vi "Analog Replay 1.0 In Place Input Write Structure.vi"(5 "Device Inputs":dbl[](array[numeric]), 7 "Last Device Inputs":dbl[](array[numeric]), 8 "error in (no error)":errorcluster, 10 "Refnum in":T3, 11 "1.0.0 Analog Replay in":T1) -> (0 "error out":errorcluster, 2 "Refnum out":T3, 3 "1.0.0 Analog Replay out":T1)   [LabVIEW 2013, in "Engine Simulation Toolkit Engine.lvlib"]
uses:
  Engine Simulation Toolkit Engine.lvlib
  Analog Replay 1.0 Input Ref.ctl
  Shared/1.0 Analog Replay Engine Data.ctl
  Shared/1.0 Analog Replay FIFO Idxs.ctl
  Shared/Engine Simulation Toolkit Shared.lvlib
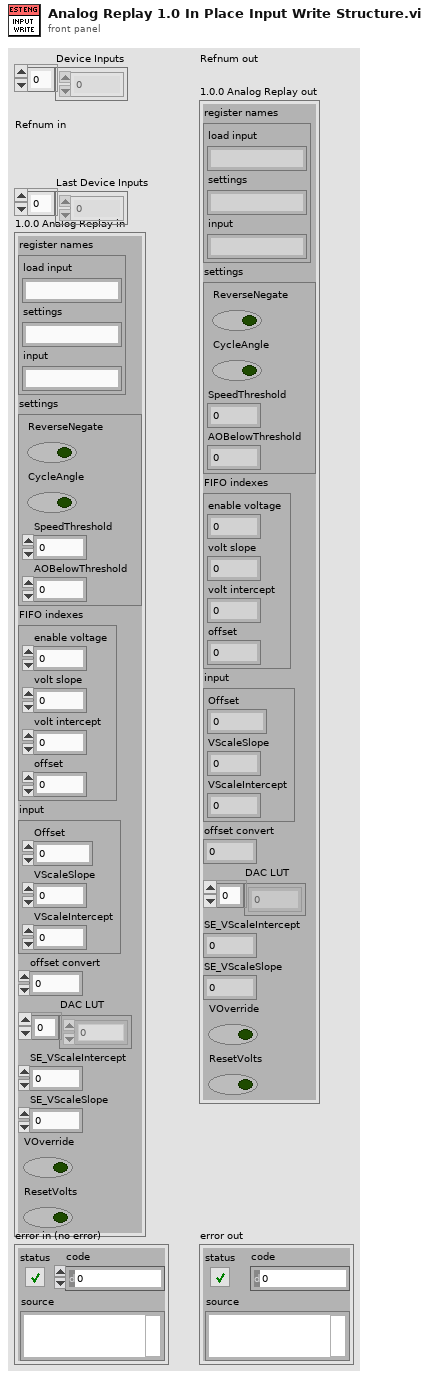
[diagram p1: front panel]
types:
  T1 = typedef "Engine Simulation Toolkit Shared.lvlib/1.0 Analog Replay Engine Data.ctl" = cluster{"register names":cluster{"load input":string, "settings":string, "input":string}, "settings":cluster{"ReverseNegate":bool, "CycleAngle":bool, "SpeedThreshold":fxp<+/-,23,2>, "AOBelowThreshold":i16}, "FIFO indexes":T2, "input":cluster{"Offset":i16, "VScaleSlope":fxp<+,18,6>, "VScaleIntercept":fxp<+/-,18,3>}, "offset convert":dbl, "DAC LUT":i16[], "SE_VScaleIntercept":fxp<+/-,18,3>, "SE_VScaleSlope":fxp<+,18,6>, "VOverride":bool, "ResetVolts":bool}
  T2 = typedef "Engine Simulation Toolkit Shared.lvlib/1.0 Analog Replay FIFO Idxs.ctl" = cluster{"enable voltage":i32, "volt slope":i32, "volt intercept":i32, "offset":i32}
  T3 = typedef "Engine Simulation Toolkit Engine.lvlib/Analog Replay 1.0 Input Ref.ctl" = refnum<k20>
  T4 = cluster{"Offset":i16, "VScaleSlope":fxp<+,18,6>, "VScaleIntercept":fxp<+/-,18,3>}
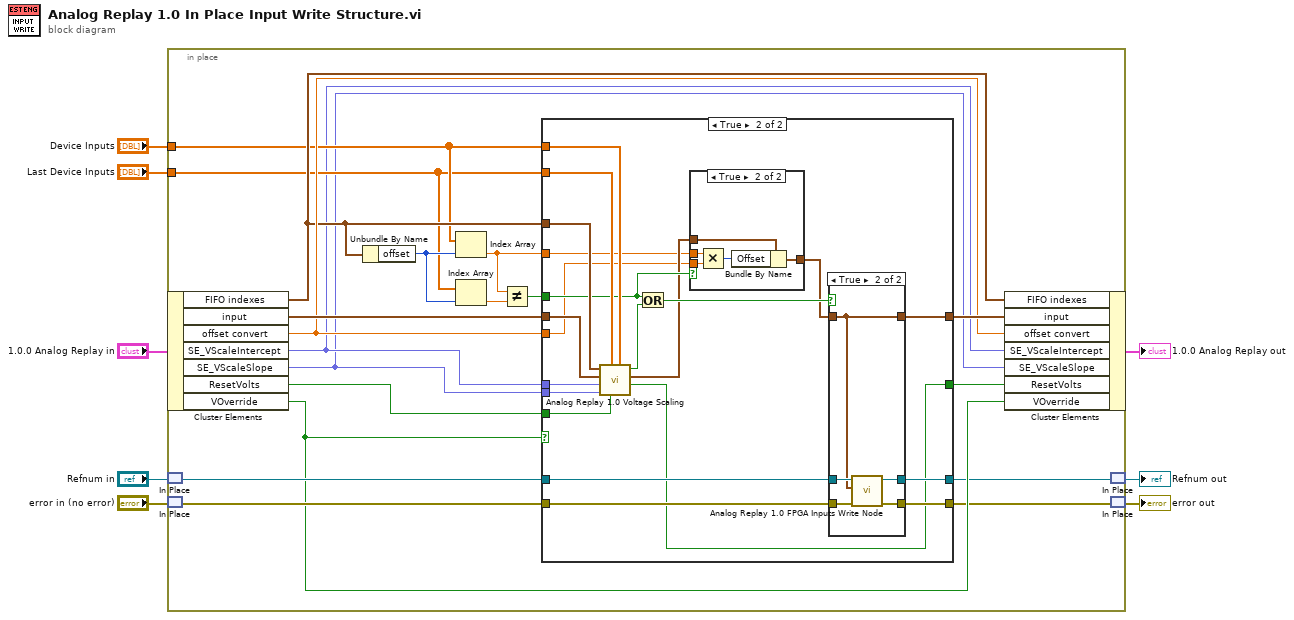
[diagram p0: block diagram]
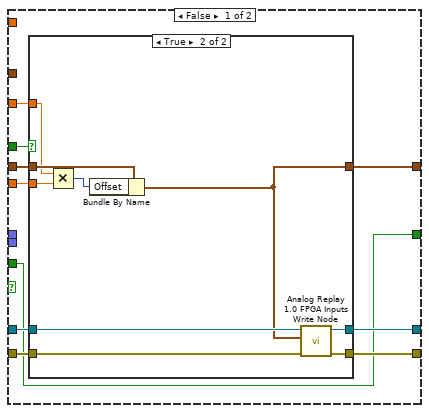
[diagram p2: hidden frame]
diagram:
  n1 = in-place {
    in-place-border: "Last Device Inputs" -> [w14]
    in-place-border: "Device Inputs" -> [w15]
    n2 = in-place-cluster #1("1.0.0 Analog Replay in") -> ("FIFO indexes"=w16:T2, "input"=w22:T4, "offset convert"=w20:dbl, "SE_VScaleIntercept"=w10:fxp<+/-,18,3>, "SE_VScaleSlope"=w9:fxp<+,18,6>, "ResetVolts"=w19:bool, "VOverride"=w25:bool)
    n3 = in-place-match #2("Refnum in") -> (w26:T3)
    n4 = in-place-match #3("error in (no error)") -> (w27:errorcluster)
    n5 = Unbundle By Name(w16) -> ("offset"=w18:i32)
    n6 = Index Array(array=w15, index=w18) -> (element=w12:dbl)
    n7 = Index Array(array=w14, index=w18) -> (element=w17:dbl)
    n8 = Not Equal?(x=w12, y=w17) -> (x != y?=w13:bool)
    n9 = case shown="True" w25 {
      tunnel: w27 -> [w37 w69]
      tunnel: w26 -> [w36 w68]
      tunnel: w16 -> [_ w61]
      tunnel: w15 -> [_ w62]
      tunnel: w14 -> [_ w63]
      tunnel: [w35 w67] -> w24
      tunnel: [w34 w66] -> w23
      tunnel: w22 -> [w33 w64]
      tunnel: w20 -> [w32 w53]
      tunnel: [w31 w65] -> w21
      tunnel: w19 -> [w28 w52]
      tunnel: w13 -> [w30 w57]
      tunnel: w12 -> [w29 w54]
      tunnel: [w28 w58] -> w11
      tunnel: w10 -> [_ w51]
      tunnel: w9 -> [_ w50]
      frame False {
        n10 = case shown="True" w30 {
          tunnel: w37 -> [w39 w42]
          tunnel: w36 -> [w40 w49]
          tunnel: [w39 w48] -> w35
          tunnel: [w40 w47] -> w34
          tunnel: w33 -> [w38 w46]
          tunnel: w29 -> [_ w45]
          tunnel: w32 -> [_ w44]
          tunnel: [w38 w41] -> w31
          frame False {
          }
          frame True {
            n11 = Multiply(x=w45, y=w44) -> (x*y=w43:i16)
            n12 = Bundle By Name(cluster=w46, "Offset"=w43) -> (w41:T4)
            n13 = call "Analog Replay 1.0 FPGA Inputs Write Node.vi"("error in (no error)"=w42, "input"=w41, "Refnum in"=w49) -> ("error out"=w48:errorcluster, "Refnum out"=w47:T3)  [unwired: 7 in]
          }
        }
      }
      frame True {
        n14 = call "Analog Replay 1.0 Voltage Scaling.vi"("Device Inputs"=w62, "reset in"=w52, "Last Device Inputs"=w63, "SE_VScaleSlope"=w50, "SE_VScaleIntercept"=w51, "input in"=w64, "FIFO indexes"=w61) -> ("reset out"=w58:bool, "input out"=w56:T4, "write"=w59:bool)  [unwired: 2 in]
        n15 = Or(x=w57, y=w59) -> (x .or. y?=w60:bool)
        n16 = case shown="True" w57 {
          tunnel: w56 -> [w70 w74]
          tunnel: [w70 w73] -> w55
          tunnel: w54 -> [_ w72]
          tunnel: w53 -> [_ w71]
          frame False {
          }
          frame True {
            n17 = Multiply(x=w72, y=w71) -> (x*y=w75:i16)
            n18 = Bundle By Name(cluster=w74, "Offset"=w75) -> (w73:T4)
          }
        }
        n19 = case shown="True" w60 {
          tunnel: w69 -> [w77 w83]
          tunnel: w68 -> [w78 w82]
          tunnel: [w77 w81] -> w67
          tunnel: [w78 w80] -> w66
          tunnel: w55 -> [w76 w79]
          tunnel: [w76 w79] -> w65
          frame False {
          }
          frame True {
            n20 = call "Analog Replay 1.0 FPGA Inputs Write Node.vi"("error in (no error)"=w83, "input"=w79, "Refnum in"=w82) -> ("error out"=w81:errorcluster, "Refnum out"=w80:T3)  [unwired: 7 in]
          }
        }
      }
    }
    n21 = in-place-cluster #1("FIFO indexes"=w16, "input"=w21, "offset convert"=w20, "SE_VScaleIntercept"=w10, "SE_VScaleSlope"=w9, "ResetVolts"=w11, "VOverride"=w25) -> (→"1.0.0 Analog Replay out":T1)
    n22 = in-place-match #2(w23) -> (→"Refnum out":T3)
    n23 = in-place-match #3(w24) -> (→"error out":errorcluster)
  }
